vi "Spindexer_Execute.vi"() -> ()   [LabVIEW 2019]
uses:
  Spindexer_Globals.vi
  Sensing/Sensor_Values.vi
  Utility_VIs/Basic_Motor_Modes.ctl
panel:
  in  "intaking_power":dbl
  in  "spin_till_position_power":dbl=0.25
  in  "ir_position_tolerance(degrees)":dbl=5.0
  in  "spindexer__ir_position_offset(degrees)":dbl
  in  "firing_velocity":dbl
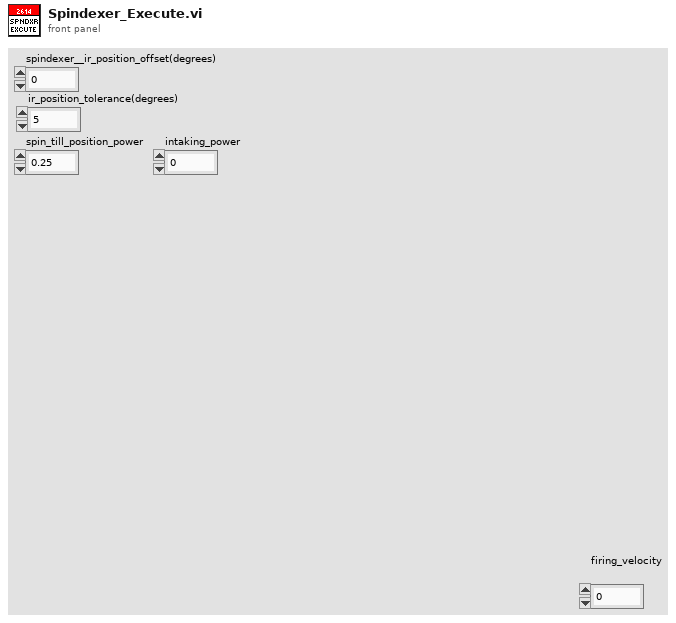
[diagram p1: front panel]
types:
  T1 = typedef "Basic_Motor_Modes.ctl" = enum16{"Percent_Voltage", "Speed_Control", "Position_Control", "Current"}
  T2 = typedef "Spindexer_Cluster.ctl" = cluster{"Throttle":dbl, "Fire?":bool, "Mode":T3}
  T3 = typedef "Spindexer_mode.ctl" = enum16{"No-Op", "Sensing", "Intaking", "Firing(Speed Control)", "Manual"}
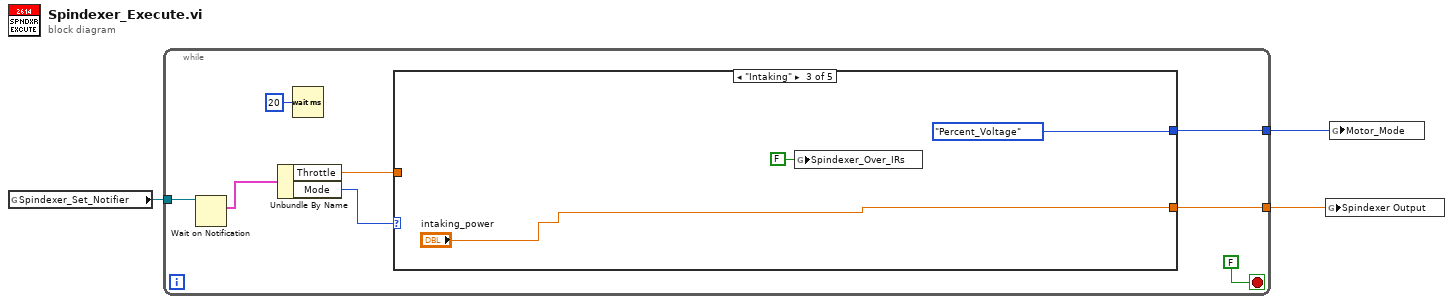
[diagram p0: block diagram]
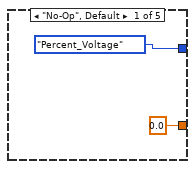
[diagram p2: hidden frame]
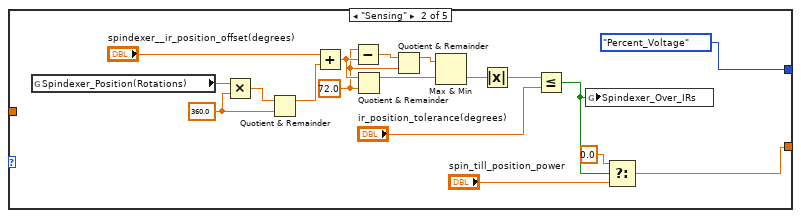
[diagram p3: hidden frame]
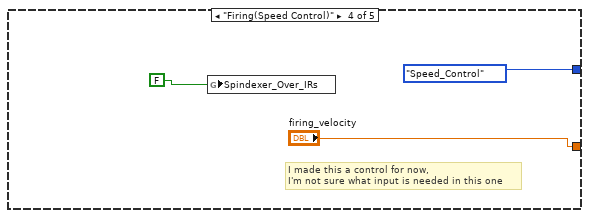
[diagram p4: hidden frame]
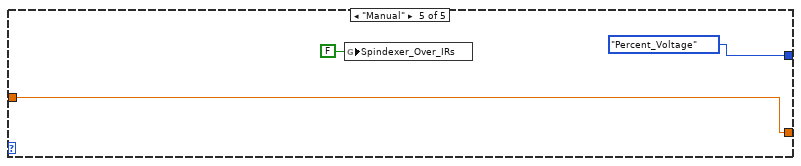
[diagram p5: hidden frame]
diagram:
  n1 = global read "Spindexer_Globals.vi" "Spindexer_Set_Notifier"() -> (w3:refnum<notifier>)
  n2 = while {
    tunnel: w3 -> [w10]
    tunnel: [w5] -> w2
    tunnel: [w6] -> w1
    stop <- FALSE stop-if-true
    n3 = Wait on Notification(notifier=w10) -> (notification=w9:T2)  [unwired: 3 in, 3 out]
    n4 = Unbundle By Name(w9) -> ("Throttle"=w7:dbl, "Mode"=w8:T3)
    n5 = Wait (ms)(milliseconds to wait=u32 20) -> ()  [unwired: 1 out]
    n6 = case shown="\"Intaking\"" w8 {
      tunnel: w7 -> [_ _ _ _ w40]
      tunnel: [0.0 ("Throttle") w30 "intaking_power" "firing_velocity" w40] -> w6
      tunnel: [Basic_Motor_Modes."Percent_Voltage" ("Basic_Motor_Mode") Basic_Motor_Modes."Percent_Voltage" ("Basic_Motor_Mode") Basic_Motor_Modes."Percent_Voltage" ("Basic_Motor_Mode") Basic_Motor_Modes."Speed_Control" ("Basic_Motor_Mode") Basic_Motor_Modes."Percent_Voltage" ("Basic_Motor_Mode")] -> w5
      frame "No-Op", Default {
      }
      frame "Sensing" {
        w22 = 72.0 ("y")
        w27 = 360.0 ("y")
        n7 = global read "Sensor_Values.vi" "Spindexer_Position(Rotations)"() -> (w29:dbl)
        n8 = Multiply(x=w29, y=w27) -> (x*y=w28:dbl)
        n9 = Quotient & Remainder(x=w28, y=w27) -> (x-y*floor(x/y)=w26:dbl)  [unwired: 1 out]
        n10 = Add(x="spindexer__ir_position_offset(degrees)", y=w26) -> (x+y=w23:dbl)
        n11 = Subtract(x=w22, y=w23) -> (x-y=w24:dbl)
        n12 = Quotient & Remainder(x=w23, y=w22) -> (x-y*floor(x/y)=w20:dbl)  [unwired: 1 out]
        n13 = Quotient & Remainder(x=w24, y=w22) -> (x-y*floor(x/y)=w21:dbl)  [unwired: 1 out]
        n14 = Max & Min(x=w21, y=w20) -> (min(x,y)=w18:dbl)  [unwired: 1 out]
        n15 = Absolute Value(x=w18) -> (abs(x)=w19:dbl)
        n16 = Less Or Equal?(x=w19, y="ir_position_tolerance(degrees)") -> (x <= y?=w16:bool)
        n17 = global write "Spindexer_Globals.vi" "Spindexer_Over_IRs"(w16) -> ()
        n18 = Select(t=0.0, s=w16, f="spin_till_position_power") -> (s? t:f=w30:dbl)
      }
      frame "Intaking" {
        n19 = global write "Spindexer_Globals.vi" "Spindexer_Over_IRs"(FALSE ("Spindexer_Over_IRs")) -> ()
      }
      frame "Firing(Speed Control)" {
        # "I made this a control for now, \nI'm not sure what input is needed in this one"
        n20 = global write "Spindexer_Globals.vi" "Spindexer_Over_IRs"(FALSE ("Spindexer_Over_IRs")) -> ()
      }
      frame "Manual" {
        n21 = global write "Spindexer_Globals.vi" "Spindexer_Over_IRs"(FALSE ("Spindexer_Over_IRs")) -> ()
      }
    }
  }
  n22 = global write "Spindexer_Globals.vi" "Spindexer Output"(w1) -> ()
  n23 = global write "Spindexer_Globals.vi" "Motor_Mode"(w2) -> ()
